vi "Cluster to Attribute Array.vi"(6 "error in (no error)":errorcluster, 9 "Cluster":variant) -> (0 "error out":errorcluster, 1 "Values":variant[](array[variant]), 2 "Names":string[](array[string]))   [LabVIEW 2017]
doc: "Converts a cluster into attribute arrays. The names of the elements of the cluster will be listed in Names, and thier corresponding values will be in Values. This VI is intended to be used in conjuction with Write Multiple Attributes.vi."
panel:
  # "LVHDF5 Toolkit\nCopyright (c) 2005-2013 by Jason D. Sommerville\nCopyright (c) 2014 by UPVI, LLC.\n\nThis use and distribution of this file is governed by the terms found in \nLICENSE.txt distributed with this toolkit and installed at\n <user.lib>\\_lvhdf5\\LICENSE.txt"
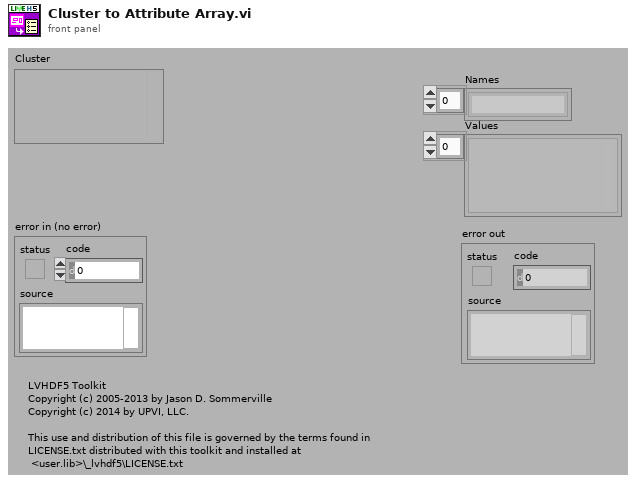
[diagram p1: front panel]
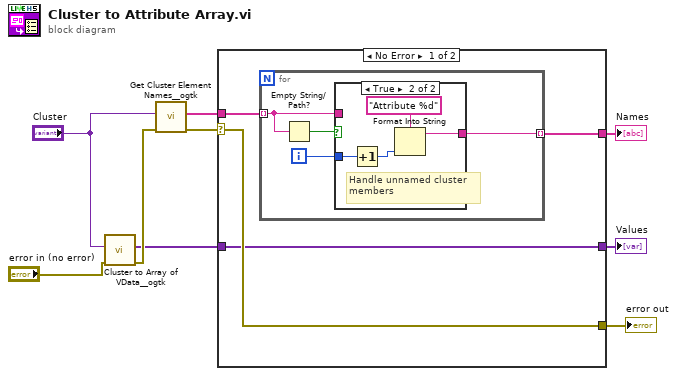
[diagram p0: block diagram]
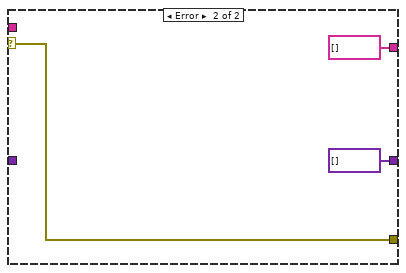
[diagram p3: hidden frame]
diagram:
  n1 = call <userlib>:"Cluster to Array of VData__ogtk.vi"("error in (no error)"="error in (no error)", "Cluster"="Cluster") -> ("error out"=w8:errorcluster, "Array of VData"=w7:variant[])  [unwired: 8 in]
  n2 = call <userlib>:"Get Cluster Element Names__ogtk.vi"("error in (no error)"=w8, "Cluster"="Cluster") -> ("error out"=w5:errorcluster, "Element Names"=w4:string[])  [unwired: 8 in]
  n3 = case shown="No Error" w5 {
    selector: w5 -> [w11 w25]
    tunnel: w7 -> [w10 _]
    tunnel: w4 -> [w13 _]
    tunnel: [w12 string[] []] -> w2
    tunnel: [w11 w25] -> w3
    tunnel: [w10 variant[] [] ("Array of VData")] -> w1
    frame No Error {
      n4 = for {
        tunnel: w13 -> [w15] mode=indexing
        tunnel: [w14] -> w12 mode=indexing
        i -> [w16]
        n5 = Empty String/Path?(string/path=w15) -> (empty?=w17:bool)
        n6 = case shown="True" w17 {
          tunnel: w16 -> [_ w22]
          tunnel: w15 -> [w18 _]
          tunnel: [w18 w19] -> w14
          frame False {
          }
          frame True {
            # "Handle unnamed cluster\nmembers"
            n7 = Increment(x=w22) -> (x+1=w21:i32)
            n8 = Format Into String(format string="Attribute %d", w21) -> (resulting string=w19:string)  [unwired: 2 in, 1 out]
          }
        }
      }
    }
    frame Error {
    }
  }
  "error out" <- w3
  "Names" <- w2
  "Values" <- w1
